vi "Get Comment Extension.vi"(8 "error in (no error)":errorcluster caption="错误输入（无错误）", 11 "Gif Image 输入":refnum<class "Gif Image.lvclass"> caption="DNL_LabVIEW Object in") -> (0 "error out":errorcluster caption="错误输出", 2 "Comment Extension":T1 {"Comment Label" format="0x%02x" items=["Image Seperator"=44, "Extension Introducer"=33, "Graphic Control Label"=249, "Comment Label"=254, "PlainText Label"=1, "Gif Trailor"=59, "Application Label"=255]; "Extension Indroducer" format="0x%02x" items=["Image Seperator"=44, "Extension Introducer"=33, "Graphic Control Label"=249, "Comment Label"=254, "PlainText Label"=1, "Gif Trailor"=59, "Application Label"=255]}, 3 "Gif Image 输出":refnum<class "Gif Image.lvclass"> caption="DNL_LabVIEW Object out")   [LabVIEW 2012, in "Picture Box Tools.lvlib" / "Gif Image.lvclass"]
uses:
  Gif Image.lvclass
  Control/Comment Extension.ctl
  Control/ID Charactor.ctl
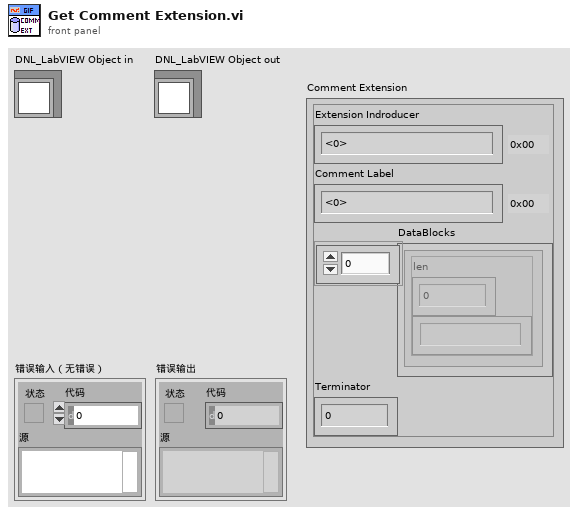
[diagram p1: front panel]
types:
  T1 = typedef "Picture Box Tools.lvlib/Gif Image.lvclass/Comment Extension.ctl" = cluster{"Extension Indroducer":T2, "Comment Label":T2, "DataBlocks":cluster{"len":u8, "字符串":string}[], "Terminator":u8}
  T2 = typedef "Picture Box Tools.lvlib/Gif Image.lvclass/ID Charactor.ctl" = u8
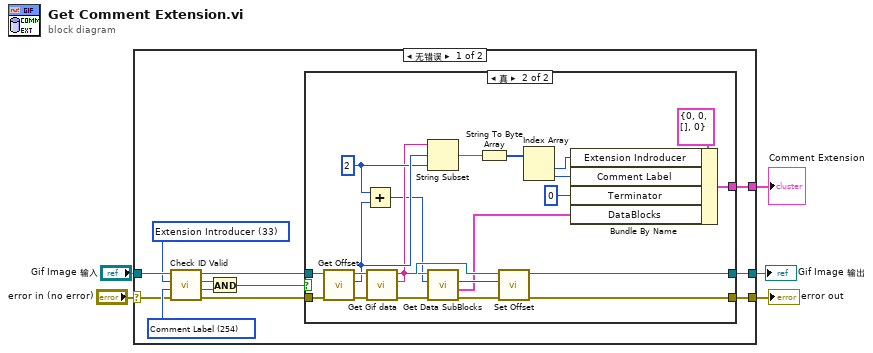
[diagram p0: block diagram]
diagram:
  n1 = case shown="无错误" "error in (no error)" {
    selector: "error in (no error)" -> [w9 w43]
    tunnel: [w7 w43] -> w4
    tunnel: [w10 _] -> w1
    tunnel: "Gif Image 输入" -> [w17 w42]
    tunnel: [w6 w42] -> w2
    frame No Error {
      w15 = T2 254 items=["Image Seperator"=44, "Extension Introducer"=33, "Graphic Control Label"=249, "Comment Label"=254, "PlainText Label"=1, "Gif Trailor"=59, "Application Label"=255] ("Label")
      w16 = T2 33 items=["Image Seperator"=44, "Extension Introducer"=33, "Graphic Control Label"=249, "Comment Label"=254, "PlainText Label"=1, "Gif Trailor"=59, "Application Label"=255] ("ID")
      n2 = call "Check ID Valid.vi"("error in (no error)"=w9, "Label"=w15, "ID"=w16, "Gif Image 输入"=w17) -> ("error out"=w8:errorcluster, "Label Valid"=w13:bool, "ID Valid"=w14:bool, "Gif Image 输出"=w11:refnum<class "Gif Image.lvclass">)  [unwired: 4 in]
      n3 = And(x=w14, y=w13) -> (x .and. y?=w12:bool)
      n4 = case shown="真" w12 {
        tunnel: w11 -> [w18 w41]
        tunnel: [_ w34] -> w10
        tunnel: w8 -> [w19 w40]
        tunnel: [w19 w30] -> w7
        tunnel: [w18 w29] -> w6
        frame False {
        }
        frame True {
          w32 = 2 ("长度（剩余）")
          n5 = call "Get Offset.vi"("error in (no error)"=w40, "Gif Image输入"=w41) -> ("error out"=w39:errorcluster, "Offset"=w33:i32, "Gif Image输出"=w38:refnum<class "Gif Image.lvclass">)  [unwired: 7 in]
          n6 = Add(x=w32, y=w33) -> (x+y=w23:i32)
          n7 = call "Get Gif data.vi"("error in (no error)"=w39, "Gif Image输入"=w38) -> ("error out"=w27:errorcluster, "Gif data"=w25:string, "Gif Image输出"=w31:refnum<class "Gif Image.lvclass">)  [unwired: 7 in]
          n8 = String Subset(string=w25, offset (0)=w33, length (rest)=w32) -> (substring=w28:string)
          n9 = call "Get Data SubBlocks.vi"("错误输入"=w27, "Offset In"=w23, "Gif data in"=w25) -> ("错误输出"=w26:errorcluster, "Data Blocks"=w20:cluster{"Len":u8, "Gif data Out":string}[], "Offset Out"=w24:i32)  [unwired: 5 in, 1 out]
          n10 = String To Byte Array(string=w28) -> (unsigned byte array=w35:u8[])
          n11 = call "Set Offset.vi"("error in (no error)"=w26, "Offset"=w24, "Gif Image输入"=w31) -> ("error out"=w30:errorcluster, "Gif Image输出"=w29:refnum<class "Gif Image.lvclass">)  [unwired: 7 in]
          n12 = Index Array(array=w35) -> (element #1=w37:u8, element #2=w36:u8)  [unwired: 2 in]
          n13 = Bundle By Name(cluster=T1 {"Extension Indroducer"=0, "Comment Label"=0, "DataBlocks"=[], "Terminator"=0} ("Comment Extension"), "Extension Indroducer"=w37, "Comment Label"=w36, "Terminator"=u8 0 ("Terminator(1)"), "DataBlocks"=w20) -> (w34:T1)
        }
      }
    }
    frame Error {
    }
  }
  "error out" <- w4
  "Gif Image 输出" <- w2
  "Comment Extension" <- w1
